vi "호출자(엄격하지않은).vi"() -> ()   [LabVIEW 2014]
panel:
  in  "signal type":T1(ring) caption="신호 타입"
  in  "frequency":dbl=10.0 caption="주파수" format="%0.2p"
  out "에러 출력":errorcluster
  out "웨이브폼 그래프":cluster{"f0":dbl, "df":dbl, "magnitude":dbl[]}
  in  "vi 경로":path
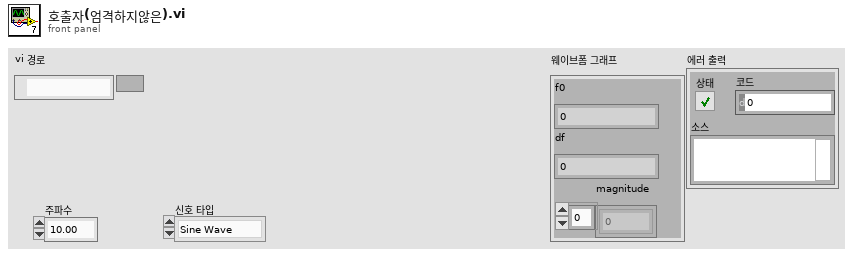
[diagram p1: front panel]
types:
  T1 = enum16{"Sine Wave", "Triangle Wave", "Square Wave", "Sawtooth Wave"}
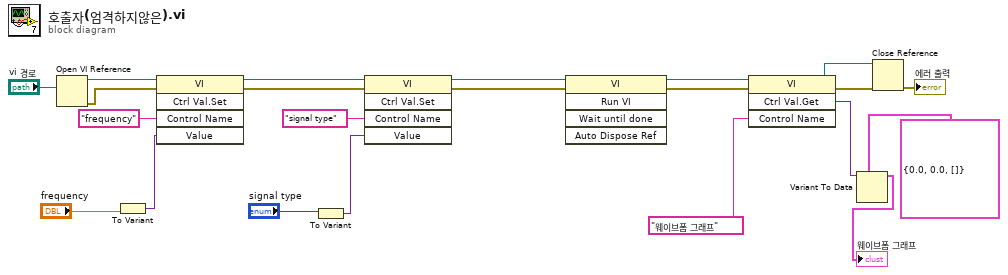
[diagram p0: block diagram]
diagram:
  n1 = Open VI Reference(vi path="vi 경로") -> (vi reference=w20:refnum<vi>, error out=w19:errorcluster)  [unwired: 5 in]
  n2 = To Variant(anything="frequency") -> (Variant=w6:variant)
  n3 = invoke class="VI" method="Ctrl Val.Set"(reference=w20, error in=w19, "Control Name"="frequency" ("컨트롤 이름"), "Value"=w6) -> (reference out=w18:refnum<vi>, error out=w17:errorcluster)  [unwired: 1 in, 3 out]
  n4 = To Variant(anything="signal type") -> (Variant=w4:variant)
  n5 = invoke class="VI" method="Ctrl Val.Set"(reference=w18, error in=w17, "Control Name"="signal type" ("컨트롤 이름"), "Value"=w4) -> (reference out=w16:refnum<vi>, error out=w15:errorcluster)  [unwired: 1 in, 3 out]
  n6 = invoke class="VI" method="Run VI"(reference=w16, error in=w15) -> (reference out=w14:refnum<vi>, error out=w13:errorcluster)  [unwired: 3 in, 3 out]
  n7 = invoke class="VI" method="Ctrl Val.Get"(reference=w14, error in=w13, "Control Name"="웨이브폼 그래프" ("컨트롤 이름")) -> (reference out=w12:refnum<vi>, error out=w11:errorcluster, "Get Control Value Variant"=w3:variant)  [unwired: 1 in, 1 out]
  n8 = Variant To Data(type=cluster{dbl, dbl, dbl[]} {0.0, 0.0, []}, Variant=w3) -> (data=→"웨이브폼 그래프":cluster{dbl, dbl, dbl[]})  [unwired: 1 in, 1 out]
  n9 = Close Reference(reference=w12, error in (no error)=w11) -> (error out=→"에러 출력":errorcluster)
